vi "StopScreen.vi"(8 "error in (no error)":errorcluster, 11 "ScreenToStop":refnum<vi>) -> (0 "error out":errorcluster)   [LabVIEW 2011]
uses:
  030 - EVENTS/EnumFgvEventCommand.ctl
  030 - EVENTS/02 - ToScreens/ToScreen.ctl
  030 - EVENTS/02 - ToScreens/ToScreensCommand.ctl
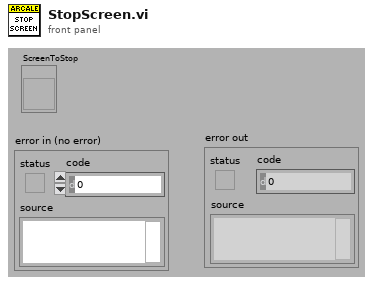
[diagram p1: front panel]
types:
  T1 = typedef "ToScreensCommand.ctl" = enum16{"Stop screen", "Stop all screens"}
  T2 = typedef "ToScreen.ctl" = cluster{"Command":T1, "Screen to stop path":path}
  T3 = typedef "EnumFgvEventCommand.ctl" = enum16{"Setup", "Cleanup", "Get"}
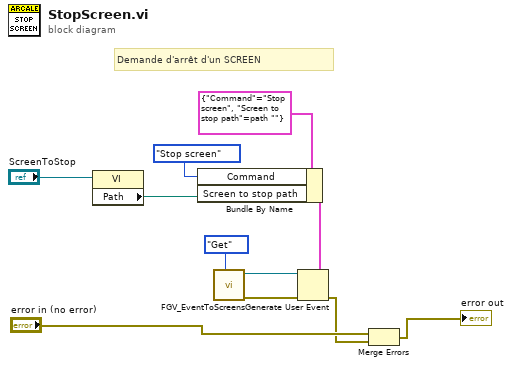
[diagram p0: block diagram]
diagram:
  # "Demande d'arrêt d'un SCREEN"
  n1 = property class="VI"(reference="ScreenToStop") -> ("Path"=w5:path)  [unwired: 1 in, 2 out]
  n2 = Bundle By Name(cluster=T2 {"Command"=enum."Stop screen", "Screen to stop path"=path ""} ("event data"), "Command"=ToScreensCommand."Stop screen", "Screen to stop path"=w5) -> (w7:T2)
  n3 = call "FGV_EventToScreens.vi"("Command"=EnumFgvEventCommand."Get") -> ("error out"=w10:errorcluster, "To Screens Event"=w9:refnum<user-event>)  [unwired: 9 in]
  n4 = Generate User Event(user event=w9, event data cluster=w7, error in=w10) -> (error out=w3:errorcluster)  [unwired: 1 out]
  n5 = Merge Errors("error in (no error)", w3) -> (→"error out":errorcluster)
